vi "Create Test Config Map.vi"(11 "VIAResult":T10 {"Test Config Data"."Test Ranking" items=["Low", "Normal", "High"]}) -> (3 "Test Config Map":T1 {"Test Config"."Test Ranking" items=["Low", "Normal", "High"]})   [LabVIEW 2023, in "VIA Results Handling.lvlib"]
doc: "Converts VIA Results Test Config Data into a map."
uses:
  VIA Results Handling.lvlib
  <vilib>/addons/analyzer/_analyzerctrls.llb/VIAnCtl Results.ctl
  <vilib>/addons/analyzer/_analyzerctrls.llb/VIAnCtl ResultsData (index).ctl
  <vilib>/addons/analyzer/_analyzerctrls.llb/VIAnCtl ResultStatus.ctl
  <vilib>/addons/analyzer/_vianresshared.llb/VIAnRes Parsed Results Data (by VI).ctl
  <vilib>/addons/analyzer/_vianresshared.llb/VIAnRes Parsed Results Data (by Test).ctl
  <vilib>/addons/analyzer/_analyzerctrls.llb/VIAnCtl Test Config Data.ctl
  <vilib>/addons/analyzer/_analyzerctrls.llb/VIAnCtl TestRanking.ctl
  <vilib>/addons/analyzer/_analyzerctrls.llb/VIAnCtl Config Control Value.ctl
  Test Config Map.ctl
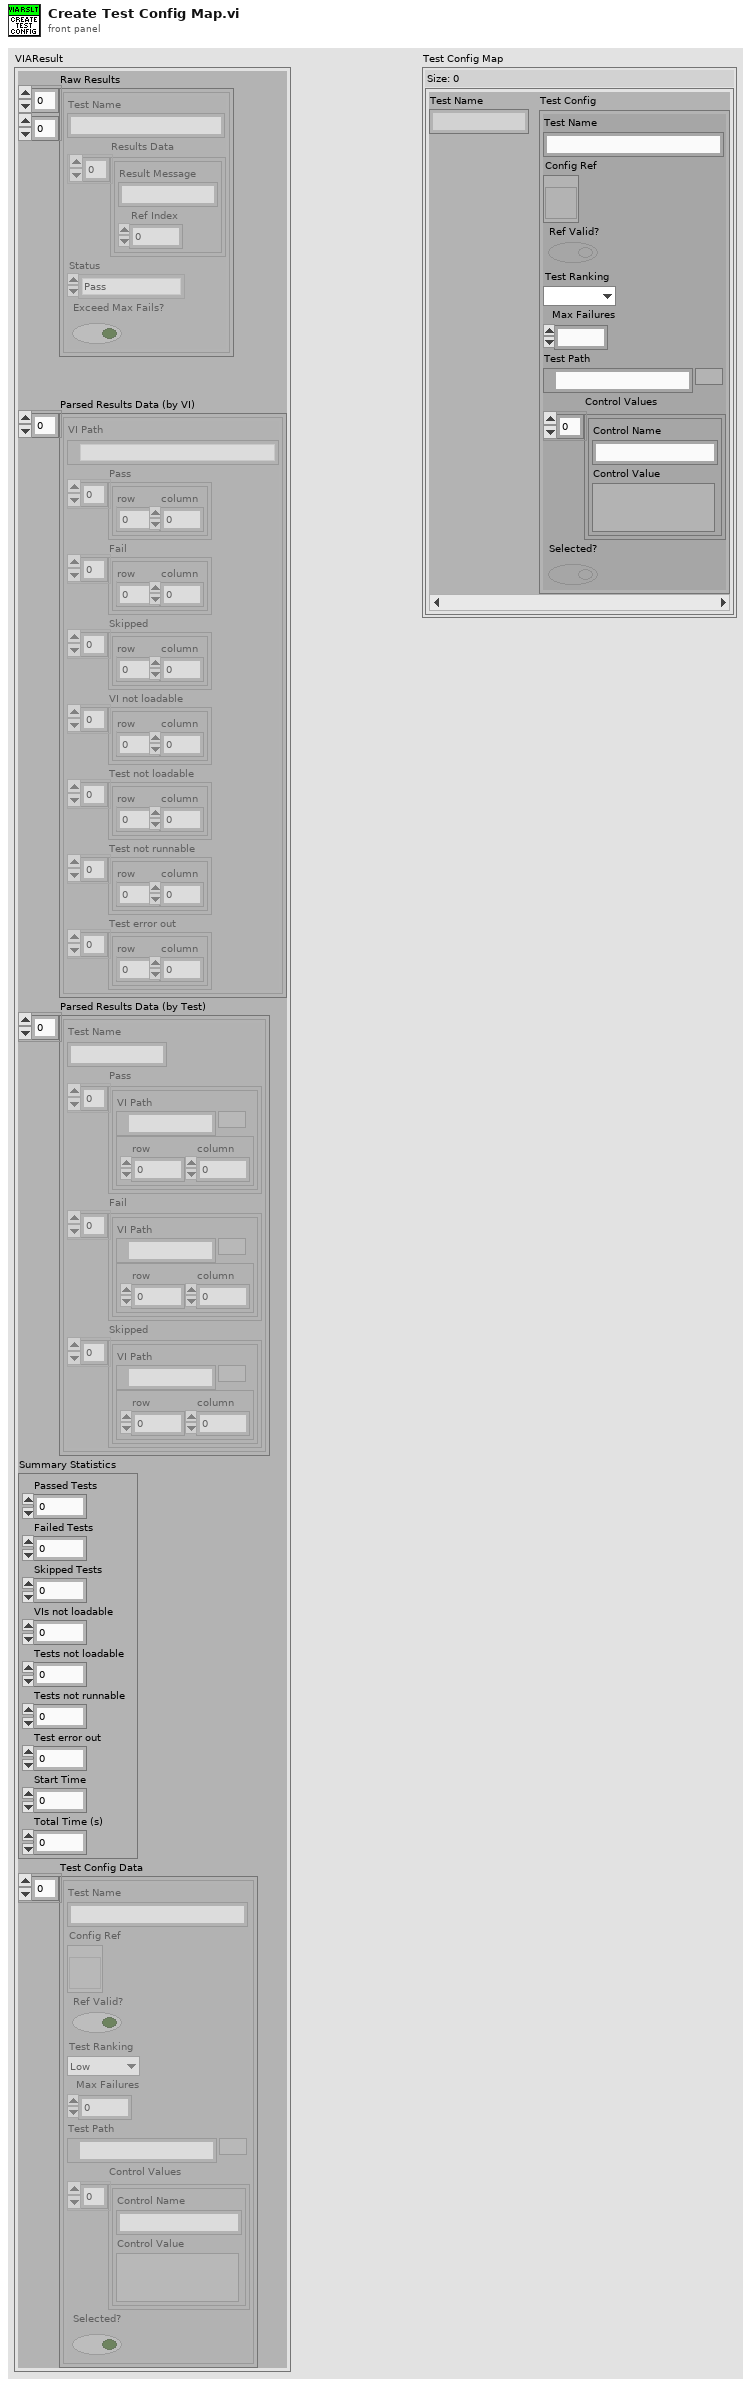
[diagram p1: front panel]
types:
  T1 = typedef "VIA Results Handling.lvlib/Test Config Map.ctl" = map{string, T2}
  T2 = typedef "VIAnCtl Test Config Data.ctl" = cluster{"Test Name":string, "Config Ref":refnum<vi>, "Ref Valid?":bool, "Test Ranking":T3, "Max Failures":u32, "Test Path":path, "Control Values":T4[], "Selected?":bool}
  T3 = typedef "VIAnCtl TestRanking.ctl" = u16
  T4 = typedef "VIAnCtl Config Control Value.ctl" = cluster{"Control Name":string, "Control Value":variant}
  T5 = typedef "VIAnCtl Results.ctl" = cluster{"Test Name":string, "Results Data":T6[], "Status":T7, "Exceed Max Fails?":bool}
  T6 = typedef "VIAnCtl ResultsData (index).ctl" = cluster{"Result Message":string, "Ref Index":i32}
  T7 = typedef "VIAnCtl ResultStatus.ctl" = enum16{"Pass", "Fail", "Skipped", "VI not loadable", "Test not loadable", "Test not runnable", "Test error out"}
  T8 = typedef "VIAnRes Parsed Results Data (by VI).ctl" = cluster{"VI Path":path, "Pass":cluster{"row":i32, "column":i32}[], "Fail":cluster{"row":i32, "column":i32}[], "Skipped":cluster{"row":i32, "column":i32}[], "VI not loadable":cluster{"row":i32, "column":i32}[], "Test not loadable":cluster{"row":i32, "column":i32}[], "Test not runnable":cluster{"row":i32, "column":i32}[], "Test error out":cluster{"row":i32, "column":i32}[]}
  T9 = typedef "VIAnRes Parsed Results Data (by Test).ctl" = cluster{"Test Name":string, "Pass":cluster{"VI Path":path, "index":cluster{"row":i32, "column":i32}}[], "Fail":cluster{"VI Path":path, "index":cluster{"row":i32, "column":i32}}[], "Skipped":cluster{"VI Path":path, "index":cluster{"row":i32, "column":i32}}[]}
  T10 = cluster{"Raw Results":T5[][], "Parsed Results Data (by VI)":T8[], "Parsed Results Data (by Test)":T9[], "Summary Statistics":cluster{"Passed Tests":i32, "Failed Tests":i32, "Skipped Tests":i32, "VIs not loadable":i32, "Tests not loadable":i32, "Tests not runnable":i32, "Test error out":i32, "Start Time":u32, "Total Time (s)":dbl}, "Test Config Data":T2[]}
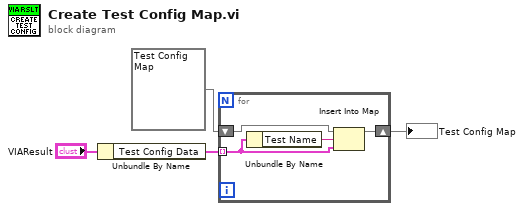
[diagram p0: block diagram]
diagram:
  n1 = Unbundle By Name("VIAResult") -> ("Test Config Data"=w4:T2[])
  n2 = for {
    tunnel: w4 -> [w5] mode=indexing
    shift-right: [w7] -> w1
    shift-left: T1 {} ("Test Ranking Map") -> [w8]
    n3 = Unbundle By Name(w5) -> ("Test Name"=w6:string)
    n4 = Insert Into Map(map in=w8, key=w6, value=w5) -> (map out=w7:T1)  [unwired: 2 out]
  }
  "Test Config Map" <- w1
